vi "Absolute Movment Command SubVi.vi"(2 "TargetPosition Y":dbl[](array[numeric]), 3 "TargetPosition X":dbl[](array[numeric]), 4 "error in":errorcluster, 5 "reference in":refnum<k24>) -> (0 "error out":errorcluster, 1 "reference out":refnum<k24>)   [LabVIEW 2017]
uses:
  Newport.XPS.CommandInterface
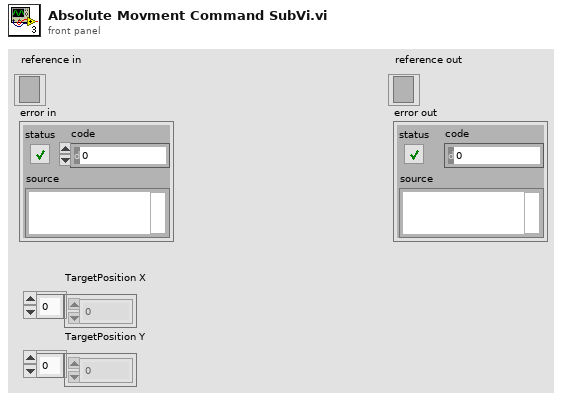
[diagram p1: front panel]
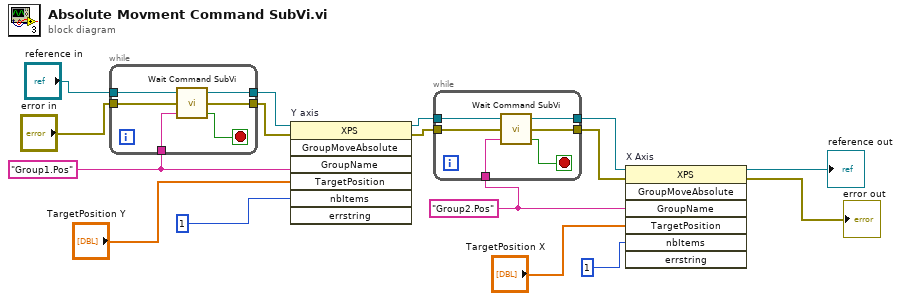
[diagram p0: block diagram]
diagram:
  w8 = "Group1.Pos"
  w5 = "Group2.Pos"
  n1 = while {
    tunnel: "reference in" -> [w22]
    tunnel: "error in" -> [w21]
    tunnel: w8 -> [w20]
    tunnel: [w18] -> w7
    tunnel: [w17] -> w6
    stop <- w19 stop-if-true
    n2 = call "Wait Command SubVi.vi"("GroupName"=w20, "error in"=w21, "reference in"=w22) -> ("Is Stop"=w19:bool, "error out"=w17:errorcluster, "reference out"=w18:refnum<k24>)
  }
  n3 = invoke on="Y axis" class="XPS" method="GroupMoveAbsolute"(reference=w7, error in=w6, "GroupName"=w8, "TargetPosition"="TargetPosition Y", "nbItems"=1) -> (reference out=w4:refnum<k24>, error out=w3:errorcluster)  [unwired: 2 in, 5 out]
  n4 = while {
    tunnel: w4 -> [w28]
    tunnel: w3 -> [w27]
    tunnel: w5 -> [w26]
    tunnel: [w24] -> w2
    tunnel: [w23] -> w1
    stop <- w25 stop-if-true
    n5 = call "Wait Command SubVi.vi"("GroupName"=w26, "error in"=w27, "reference in"=w28) -> ("Is Stop"=w25:bool, "error out"=w23:errorcluster, "reference out"=w24:refnum<k24>)
  }
  n6 = invoke on="X Axis" class="XPS" method="GroupMoveAbsolute"(reference=w2, error in=w1, "GroupName"=w5, "TargetPosition"="TargetPosition X", "nbItems"=1) -> (reference out=→"reference out":refnum<k24>, error out=→"error out":errorcluster)  [unwired: 2 in, 5 out]
